vi "Autonomous Load.vi"(0 "Number of Commands":i32, 5 "Subsystems":string[](array[string]), 7 "Commands":string[](array[string]), 9 "Inputs":string[](array[string]), 11 "error in":errorcluster) -> (4 "Queue Key":refnum<queue>, 8 "Autonomous Queue":refnum<queue>, 15 "errror out":errorcluster)   [LabVIEW 2016]
uses:
  Drive/Drive Control Type.ctl
  Intake/Intake Control Type.ctl
  Rotation/Rotation Control Type.ctl
  Robot Subsystems.ctl
  Drive/Drive Notifier.ctl
  Climb/Climb Notifier.ctl
  Climb/Climb Control Type.ctl
  Intake/Intake Notifier.ctl
  Rotation/Rotation Notifier.ctl
  Queue Key Data.ctl
  Drive/Drive Globals.vi
  Intake/Intake Globals.vi
  Rotation/Rotation Globals.vi
panel:
  in  "Rotation Control List":T1
  in  "Intake Control List":T2
  out "Subsystem":string
  in  "Drive Control List":T3
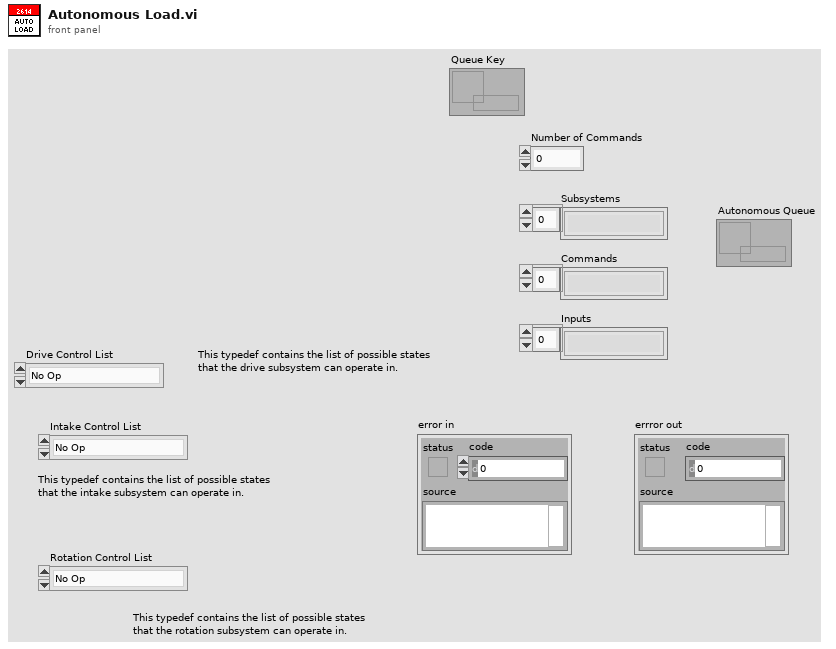
[diagram p1: front panel]
types:
  T1 = typedef "Rotation Control Type.ctl" = enum16{"No Op", "Up", "Down", "Control Up", "Control Down", "Gear Down", "Gear Up"}
  T2 = typedef "Intake Control Type.ctl" = enum16{"No Op", "In", "Out"}
  T3 = typedef "Drive Control Type.ctl" = enum16{"No Op", "Fieldcentric", "Robotcentric", "Reset Wheel Position", "Reset Gyro Value", "Turn to Angle", "Drive For Time"}
  T4 = typedef "Queue Key Data.ctl" = cluster{"Operation Notifier":refnum<notifier>, "Subsystem":string, "Concurrent":bool}
  T5 = typedef "Robot Subsystems.ctl" = cluster{"Drive Notifier":T6, "Climb Notifier":T7, "Intake Notifier":T9, "Rotation Notifier":T10}
  T6 = typedef "Drive Notifier.ctl" = cluster{"Parameter 1":dbl, "Parameter 2":dbl, "Parameter 3":dbl, "Drive Control List":T3, "Parameter 4":dbl, "Gear Angle":dbl, "Parameter 6":dbl, "Parameter 7":dbl, "Parameter 8":dbl, "Parameter 9":dbl, "Robotcentric":bool, "Reset Gyro":bool, "Reset Wheels":bool, "Turn to Gear Left":bool, "Turn to Gear Center":bool, "Turn to Gear Right":bool, "Half Power":bool, "Drive Notifier":refnum<notifier>, "Step":i32}
  T7 = typedef "Climb Notifier.ctl" = cluster{"Up":bool, "Down":bool, "Climb Control List":T8}
  T8 = typedef "Climb Control Type.ctl" = enum16{"No Op", "Up", "Down"}
  T9 = typedef "Intake Notifier.ctl" = cluster{"In":bool, "Out":bool, "Intake Control List":T2, "Parameter 1":dbl, "Parameter 2":dbl, "Intake Notifier":refnum<notifier>, "Step":i32}
  T10 = typedef "Rotation Notifier.ctl" = cluster{"Up":bool, "Down":bool, "Rotation Control List":T1, "Control Down":bool, "Manual":bool, "Parameter 1":dbl, "Parameter 2":dbl, "Rotation Notifier":refnum<notifier>, "Step":i32}
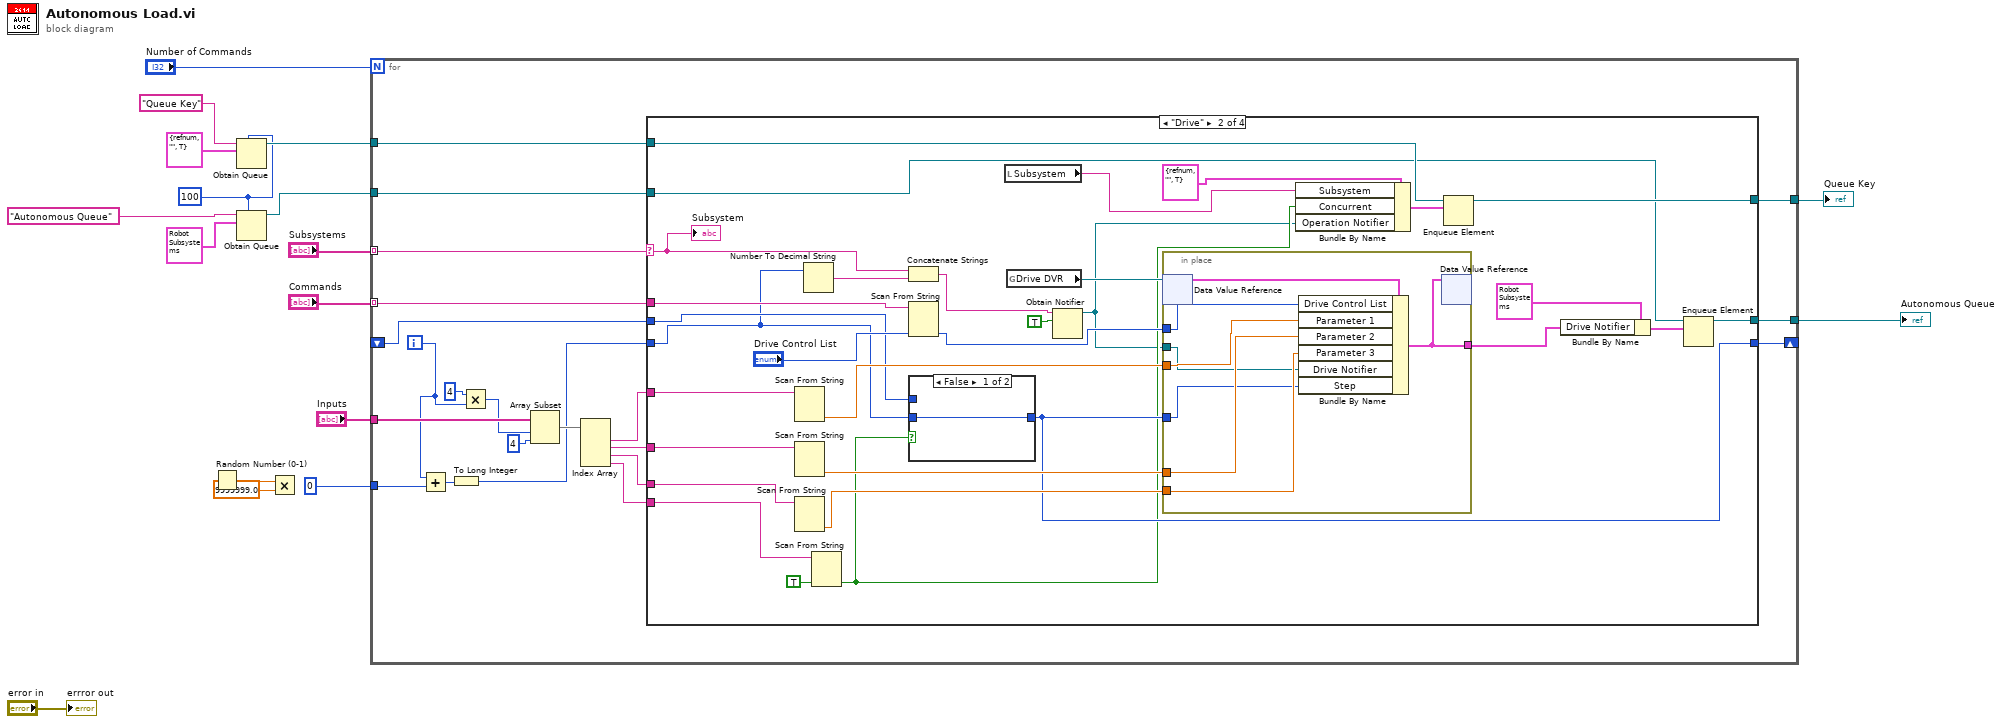
[diagram p0: block diagram]
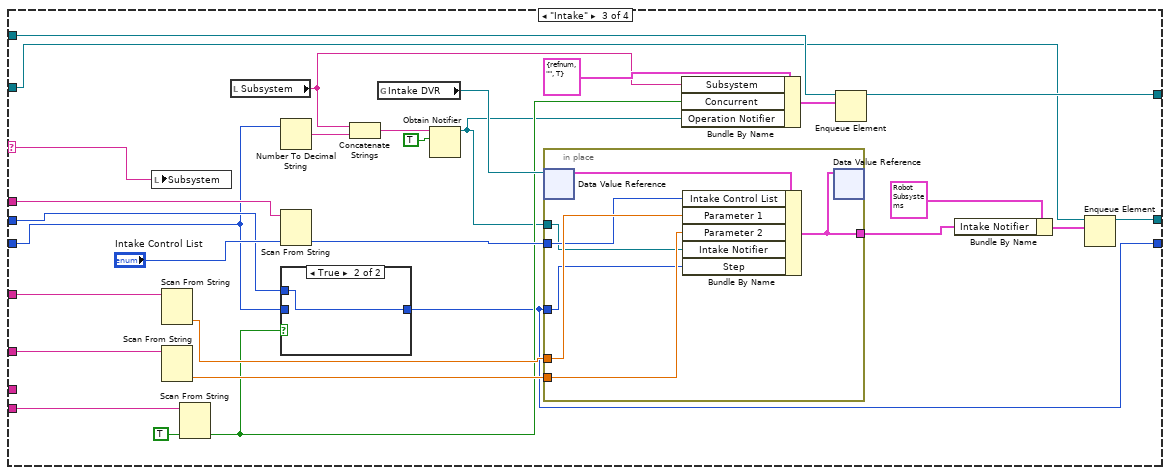
[diagram p4: hidden frame]
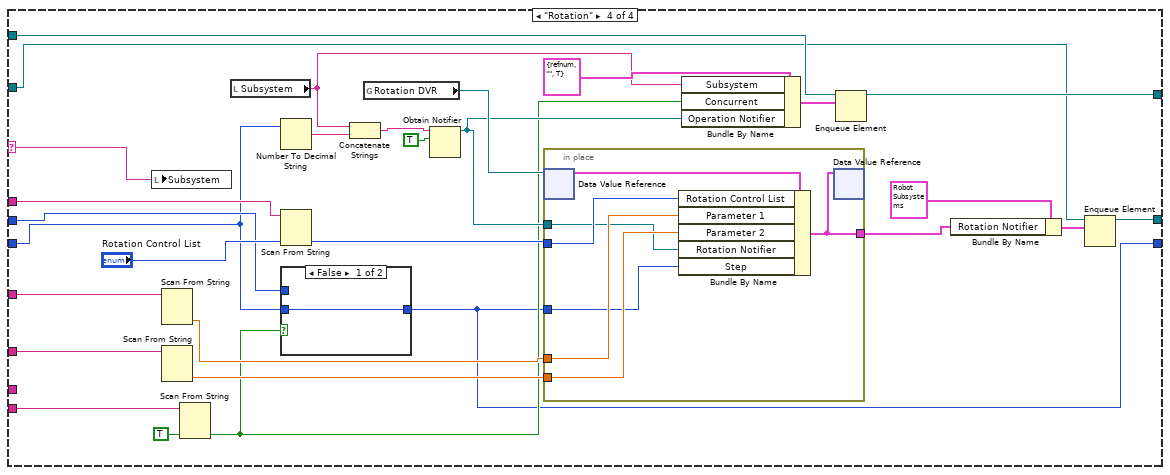
[diagram p6: hidden frame]
diagram:
  w7 = 100 ("max queue size (-1, unlimited)")
  n1 = Random Number (0-1)() -> (number: 0 to 1=w3:dbl)
  n2 = Obtain Queue(max queue size (-1, unlimited)=w7, name (unnamed)="Queue Key", element data type=T4 {"Operation Notifier"=refnum, "Subsystem"="", "Concurrent"=TRUE} ("Queue Key Data")) -> (queue out=w15:refnum<queue>)  [unwired: 2 in, 2 out]
  n3 = Obtain Queue(max queue size (-1, unlimited)=w7, name (unnamed)="Autonomous Queue", element data type=T5 {"Drive Notifier"={"Parameter 1"=0.0, "Parameter 2"=0.0, "Parameter 3"=0.0, "Drive Control List"=enum."No Op", "Parameter 4"=0.0, "Gear Angle"=0.0, "Parameter 6"=0.0, "Parameter 7"=0.0, "Parameter 8"=0.0, "Parameter 9"=0.0, "Robotcentric"=FALSE, "Reset Gyro"=FALSE, "Reset Wheels"=FALSE, "Turn to Gear Left"=FALSE, "Turn to Gear Center"=FALSE, "Turn to Gear Right"=FALSE, "Half Power"=FALSE, "Drive Notifier"=refnum, "Step"=0}, "Climb Notifier"={"Up"=FALSE, "Down"=FALSE, "Climb Control List"=enum."No Op"}, "Intake Notifier"={"In"=FALSE, "Out"=FALSE, "Intake Control List"=enum."No Op", "Parameter 1"=0.0, "Parameter 2"=0.0, "Intake Notifier"=refnum, "Step"=0}, "Rotation Notifier"={"Up"=FALSE, "Down"=FALSE, "Rotation Control List"=enum."No Op", "Control Down"=FALSE, "Manual"=FALSE, "Parameter 1"=0.0, "Parameter 2"=0.0, "Rotation Notifier"=refnum, "Step"=0}} ("Robot Subsytems")) -> (queue out=w8:refnum<queue>)  [unwired: 2 in, 2 out]
  n4 = Multiply(x=w3, y=9999999.0) -> ()  [unwired: 1 out]
  n5 = for {
    N: "Number of Commands" -> [_]
    tunnel: w15 -> [w38]
    tunnel: "Subsystems" -> [w37] mode=indexing
    tunnel: "Commands" -> [w36] mode=indexing
    tunnel: "Inputs" -> [w31]
    tunnel: [w26] -> w4
    tunnel: w8 -> [w25]
    tunnel: [w24] -> w6
    shift-right: [w22] -> _
    shift-left: _ -> [w23]
    tunnel: 0 ("y") -> [w18]
    i -> [w21]
    n6 = Add(x=w21, y=w18) -> (x+y=w20:i32)
    n7 = To Long Integer(number=w20) -> (32bit integer=w19:i32)
    n8 = Multiply(x=4, y=w21) -> (x*y=w28:i32)
    n9 = Array Subset(array=w31, index=w28, length=4) -> (w30:string[])
    n10 = Index Array(array=w30) -> (element #1=w35:string, element #2=w34:string, element #3=w33:string, element #4=w32:string)  [unwired: 4 in]
    n11 = case shown="\"Drive\"" w37 {
      selector: w37 -> [_ w52 w105 w143]
      tunnel: w38 -> [w40 w68 w108 w146]
      tunnel: w36 -> [_ w62 w101 w139]
      tunnel: w35 -> [_ w61 w100 w138]
      tunnel: w34 -> [_ w60 w99 w137]
      tunnel: w33 -> [_ w59 _ _]
      tunnel: w32 -> [_ w58 w98 w121]
      tunnel: [w41 w54 w96 w135] -> w24
      tunnel: [w40 w56 w95 w134] -> w26
      tunnel: w25 -> [w41 w55 w94 w133]
      tunnel: w23 -> [_ w51 w92 w131]
      tunnel: w19 -> [w39 w42 w89 w128]
      tunnel: [w39 w50 w83 w122] -> w22
      frame "No Op", Default {
      }
      frame "Drive" {
        n12 = Scan From String(input string=w61) -> (output 1=w71:dbl)  [unwired: 4 in, 3 out]
        n13 = Scan From String(input string=w60) -> (output 1=w70:dbl)  [unwired: 4 in, 3 out]
        n14 = Scan From String(input string=w59) -> (output 1=w63:dbl)  [unwired: 4 in, 3 out]
        n15 = Number To Decimal String(number=w42) -> (decimal integer string=w43:string)  [unwired: 1 in]
        n16 = Scan From String(input string=w58, default 1=TRUE) -> (output 1=w46:bool)  [unwired: 3 in, 3 out]
        n17 = Concatenate Strings(w52, w43) -> (w49:string)
        n18 = Scan From String(input string=w62, default 1="Drive Control List") -> (output 1=w72:T3)  [unwired: 3 in, 3 out]
        n19 = case shown="False" w46 {
          tunnel: [w73 w74] -> w50
          tunnel: w51 -> [_ w74]
          tunnel: w42 -> [w73 _]
          frame False {
          }
          frame True {
          }
        }
        n20 = local read "Subsystem"() -> (w47:string)
        n21 = global read "Drive Globals.vi" "Drive DVR"() -> (w67:refnum<data-value>)
        n22 = Obtain Notifier(name (unnamed)=w49, notification data type=TRUE) -> (notifier out=w45:refnum<notifier>)  [unwired: 2 in, 2 out]
        n23 = in-place {
          in-place-border: w72 -> [w78]
          in-place-border: [w81] -> w69
          in-place-border: w71 -> [w80]
          in-place-border: w70 -> [w79]
          in-place-border: w63 -> [w77]
          in-place-border: w45 -> [w76]
          in-place-border: w50 -> [w75]
          n24 = in-place-dvr #1(w67) -> (w82:T6)  [unwired: 1 out]
          n25 = Bundle By Name(cluster=w82, "Drive Control List"=w78, "Parameter 1"=w80, "Parameter 2"=w79, "Parameter 3"=w77, "Drive Notifier"=w76, "Step"=w75) -> (w81:T6)
          n26 = in-place-dvr #1(w81) -> ()  [unwired: 2 out]
        }
        n27 = Bundle By Name(cluster=T4 {"Operation Notifier"=refnum, "Subsystem"="", "Concurrent"=TRUE} ("Queue Key Data"), "Subsystem"=w47, "Concurrent"=w46, "Operation Notifier"=w45) -> (w44:T4)
        n28 = Enqueue Element(queue=w68, element=w44) -> (queue out=w56:refnum<queue>)  [unwired: 2 in, 2 out]
        n29 = Bundle By Name(cluster=T5 {"Drive Notifier"={"Parameter 1"=0.0, "Parameter 2"=0.0, "Parameter 3"=0.0, "Drive Control List"=enum."No Op", "Parameter 4"=0.0, "Gear Angle"=0.0, "Parameter 6"=0.0, "Parameter 7"=0.0, "Parameter 8"=0.0, "Parameter 9"=0.0, "Robotcentric"=FALSE, "Reset Gyro"=FALSE, "Reset Wheels"=FALSE, "Turn to Gear Left"=FALSE, "Turn to Gear Center"=FALSE, "Turn to Gear Right"=FALSE, "Half Power"=FALSE, "Drive Notifier"=refnum, "Step"=0}, "Climb Notifier"={"Up"=FALSE, "Down"=FALSE, "Climb Control List"=enum."No Op"}, "Intake Notifier"={"In"=FALSE, "Out"=FALSE, "Intake Control List"=enum."No Op", "Parameter 1"=0.0, "Parameter 2"=0.0, "Intake Notifier"=refnum, "Step"=0}, "Rotation Notifier"={"Up"=FALSE, "Down"=FALSE, "Rotation Control List"=enum."No Op", "Control Down"=FALSE, "Manual"=FALSE, "Parameter 1"=0.0, "Parameter 2"=0.0, "Rotation Notifier"=refnum, "Step"=0}} ("Robot Subsytems"), "Drive Notifier"=w69) -> (w65:T5)
        n30 = Enqueue Element(queue=w55, element=w65) -> (queue out=w54:refnum<queue>)  [unwired: 2 in, 2 out]
        "Subsystem" <- w52
      }
      frame "Intake" {
        n31 = local write "Subsystem"(w105) -> ()
        n32 = Scan From String(input string=w100) -> (output 1=w110:dbl)  [unwired: 4 in, 3 out]
        n33 = Scan From String(input string=w99) -> (output 1=w109:dbl)  [unwired: 4 in, 3 out]
        n34 = Scan From String(input string=w98, default 1=TRUE) -> (output 1=w85:bool)  [unwired: 3 in, 3 out]
        n35 = local read "Subsystem"() -> (w86:string)
        n36 = Number To Decimal String(number=w89) -> (decimal integer string=w90:string)  [unwired: 1 in]
        n37 = Scan From String(input string=w101, default 1="Intake Control List") -> (output 1=w111:T2)  [unwired: 3 in, 3 out]
        n38 = case shown="True" w85 {
          tunnel: [w112 w113] -> w83
          tunnel: w92 -> [_ w113]
          tunnel: w89 -> [w112 _]
          frame False {
          }
          frame True {
          }
        }
        n39 = Concatenate Strings(w86, w90) -> (w91:string)
        n40 = global read "Intake Globals.vi" "Intake DVR"() -> (w104:refnum<data-value>)
        n41 = Obtain Notifier(name (unnamed)=w91, notification data type=TRUE) -> (notifier out=w84:refnum<notifier>)  [unwired: 2 in, 2 out]
        n42 = in-place {
          in-place-border: w111 -> [w116]
          in-place-border: [w119] -> w102
          in-place-border: w110 -> [w118]
          in-place-border: w109 -> [w117]
          in-place-border: w84 -> [w115]
          in-place-border: w83 -> [w114]
          n43 = in-place-dvr #2(w104) -> (w120:T9)  [unwired: 1 out]
          n44 = Bundle By Name(cluster=w120, "Intake Control List"=w116, "Parameter 1"=w118, "Parameter 2"=w117, "Intake Notifier"=w115, "Step"=w114) -> (w119:T9)
          n45 = in-place-dvr #2(w119) -> ()  [unwired: 2 out]
        }
        n46 = Bundle By Name(cluster=T4 {"Operation Notifier"=refnum, "Subsystem"="", "Concurrent"=TRUE} ("Queue Key Data"), "Subsystem"=w86, "Concurrent"=w85, "Operation Notifier"=w84) -> (w87:T4)
        n47 = Enqueue Element(queue=w108, element=w87) -> (queue out=w95:refnum<queue>)  [unwired: 2 in, 2 out]
        n48 = Bundle By Name(cluster=T5 {"Drive Notifier"={"Parameter 1"=0.0, "Parameter 2"=0.0, "Parameter 3"=0.0, "Drive Control List"=enum."No Op", "Parameter 4"=0.0, "Gear Angle"=0.0, "Parameter 6"=0.0, "Parameter 7"=0.0, "Parameter 8"=0.0, "Parameter 9"=0.0, "Robotcentric"=FALSE, "Reset Gyro"=FALSE, "Reset Wheels"=FALSE, "Turn to Gear Left"=FALSE, "Turn to Gear Center"=FALSE, "Turn to Gear Right"=FALSE, "Half Power"=FALSE, "Drive Notifier"=refnum, "Step"=0}, "Climb Notifier"={"Up"=FALSE, "Down"=FALSE, "Climb Control List"=enum."No Op"}, "Intake Notifier"={"In"=FALSE, "Out"=FALSE, "Intake Control List"=enum."No Op", "Parameter 1"=0.0, "Parameter 2"=0.0, "Intake Notifier"=refnum, "Step"=0}, "Rotation Notifier"={"Up"=FALSE, "Down"=FALSE, "Rotation Control List"=enum."No Op", "Control Down"=FALSE, "Manual"=FALSE, "Parameter 1"=0.0, "Parameter 2"=0.0, "Rotation Notifier"=refnum, "Step"=0}} ("Robot Subsytems"), "Intake Notifier"=w102) -> (w107:T5)
        n49 = Enqueue Element(queue=w94, element=w107) -> (queue out=w96:refnum<queue>)  [unwired: 2 in, 2 out]
      }
      frame "Rotation" {
        n50 = local write "Subsystem"(w143) -> ()
        n51 = Scan From String(input string=w138) -> (output 1=w148:dbl)  [unwired: 4 in, 3 out]
        n52 = Scan From String(input string=w137) -> (output 1=w147:dbl)  [unwired: 4 in, 3 out]
        n53 = Scan From String(input string=w121, default 1=TRUE) -> (output 1=w124:bool)  [unwired: 3 in, 3 out]
        n54 = local read "Subsystem"() -> (w123:string)
        n55 = Number To Decimal String(number=w128) -> (decimal integer string=w129:string)  [unwired: 1 in]
        n56 = Scan From String(input string=w139, default 1="Rotation Control List") -> (output 1=w149:T1)  [unwired: 3 in, 3 out]
        n57 = case shown="False" w124 {
          tunnel: [w150 w151] -> w122
          tunnel: w131 -> [_ w151]
          tunnel: w128 -> [w150 _]
          frame False {
          }
          frame True {
          }
        }
        n58 = Concatenate Strings(w123, w129) -> (w130:string)
        n59 = global read "Rotation Globals.vi" "Rotation DVR"() -> (w142:refnum<data-value>)
        n60 = Obtain Notifier(name (unnamed)=w130, notification data type=TRUE) -> (notifier out=w125:refnum<notifier>)  [unwired: 2 in, 2 out]
        n61 = in-place {
          in-place-border: w149 -> [w154]
          in-place-border: [w157] -> w141
          in-place-border: w148 -> [w156]
          in-place-border: w147 -> [w155]
          in-place-border: w125 -> [w153]
          in-place-border: w122 -> [w152]
          n62 = in-place-dvr #3(w142) -> (w158:T10)  [unwired: 1 out]
          n63 = Bundle By Name(cluster=w158, "Rotation Control List"=w154, "Parameter 1"=w156, "Parameter 2"=w155, "Rotation Notifier"=w153, "Step"=w152) -> (w157:T10)
          n64 = in-place-dvr #3(w157) -> ()  [unwired: 2 out]
        }
        n65 = Bundle By Name(cluster=T4 {"Operation Notifier"=refnum, "Subsystem"="", "Concurrent"=TRUE} ("Queue Key Data"), "Subsystem"=w123, "Concurrent"=w124, "Operation Notifier"=w125) -> (w126:T4)
        n66 = Enqueue Element(queue=w146, element=w126) -> (queue out=w134:refnum<queue>)  [unwired: 2 in, 2 out]
        n67 = Bundle By Name(cluster=T5 {"Drive Notifier"={"Parameter 1"=0.0, "Parameter 2"=0.0, "Parameter 3"=0.0, "Drive Control List"=enum."No Op", "Parameter 4"=0.0, "Gear Angle"=0.0, "Parameter 6"=0.0, "Parameter 7"=0.0, "Parameter 8"=0.0, "Parameter 9"=0.0, "Robotcentric"=FALSE, "Reset Gyro"=FALSE, "Reset Wheels"=FALSE, "Turn to Gear Left"=FALSE, "Turn to Gear Center"=FALSE, "Turn to Gear Right"=FALSE, "Half Power"=FALSE, "Drive Notifier"=refnum, "Step"=0}, "Climb Notifier"={"Up"=FALSE, "Down"=FALSE, "Climb Control List"=enum."No Op"}, "Intake Notifier"={"In"=FALSE, "Out"=FALSE, "Intake Control List"=enum."No Op", "Parameter 1"=0.0, "Parameter 2"=0.0, "Intake Notifier"=refnum, "Step"=0}, "Rotation Notifier"={"Up"=FALSE, "Down"=FALSE, "Rotation Control List"=enum."No Op", "Control Down"=FALSE, "Manual"=FALSE, "Parameter 1"=0.0, "Parameter 2"=0.0, "Rotation Notifier"=refnum, "Step"=0}} ("Robot Subsytems"), "Rotation Notifier"=w141) -> (w145:T5)
        n68 = Enqueue Element(queue=w133, element=w145) -> (queue out=w135:refnum<queue>)  [unwired: 2 in, 2 out]
      }
    }
  }
  "Autonomous Queue" <- w6
  "Queue Key" <- w4
  "errror out" <- "error in"
